vi "CalibrationDialog.vi"() -> (0 "OK 2":bool, 1 "Curve Number":i32=7 min=6 max=31, 2 "Sensor Type display":i32)   [LabVIEW 2020]
panel:
  in  "Sensor Type":i32(ring) items=["Carbon Glass", "Platinum", "Diode"]
  in  "Cancel":bool
  in  "OK":bool
  in  "LakeShore Curve Number:":i32=7 min=6 max=31
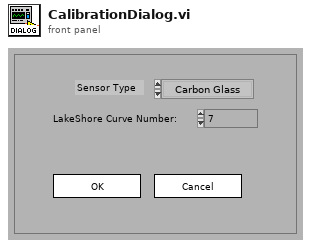
[diagram p1: front panel]
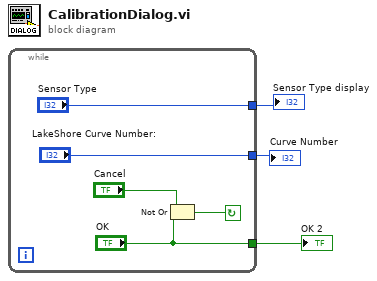
[diagram p0: block diagram]
diagram:
  n1 = while {
    tunnel: ["Sensor Type"] -> w1
    tunnel: ["LakeShore Curve Number:"] -> w2
    tunnel: ["OK"] -> w3
    stop <- w6 continue-if-true
    n2 = Not Or(1:"OK", 2:"Cancel") -> (0:w6:bool)
  }
  "OK 2" <- w3
  "Sensor Type display" <- w1
  "Curve Number" <- w2
